vi "Analysis.Selection.Create.vi"(8 "error in (no error)":errorcluster, 9 "Name":string, 10 "Analysis Options":T2, 11 "Item Ref in":T1 format="%.0x") -> (0 "error out":errorcluster)   [LabVIEW 2015, in "Fuel Injection Addon System Explorer.lvlib"]
uses:
  Fuel Injection Addon System Explorer.lvlib
  Shared/Types/Analysis.Channels.Select.ctl
  <vilib>/NI Veristand/Custom Device API/Custom Device Item Ref.ctl
  Shared/Constants.vi
  <vilib>/NI Veristand/Custom Device Tools/Custom Device Utility Library/NI VeriStand - Search for All Items by GUID.vi
  <vilib>/NI VeriStand/Custom Device API/Custom Device API.lvlib
  <vilib>/NI Veristand/Custom Device Tools/Custom Device Utility Library/Custom Device Utility Library.lvlib
  Shared/Fuel Injection Addon Shared.lvlib
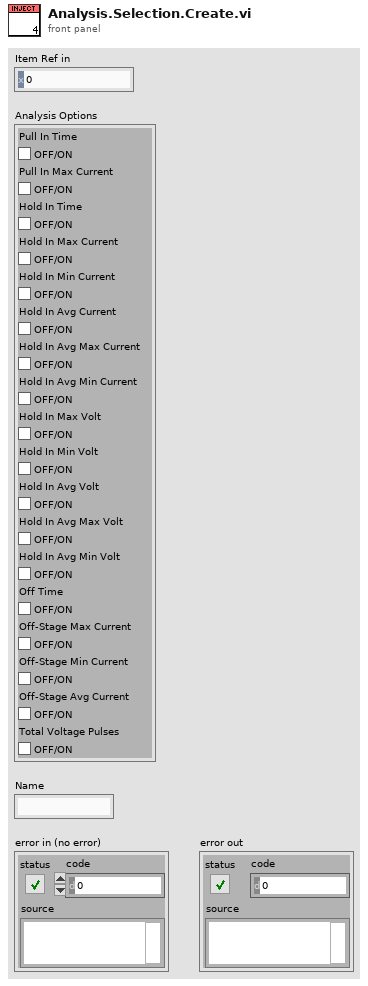
[diagram p1: front panel]
types:
  T1 = typedef "Custom Device API.lvlib/Custom Device Item Ref.ctl" = u64
  T2 = typedef "Fuel Injection Addon Shared.lvlib/Analysis.Channels.Select.ctl" = cluster{"Pull In Time":bool, "Pull In Max Current":bool, "Hold In Time":bool, "Hold In Max Current":bool, "Hold In Min Current":bool, "Hold In Avg Current":bool, "Hold In Avg Max Current":bool, "Hold In Avg Min Current":bool, "Hold In Max Volt":bool, "Hold In Min Volt":bool, "Hold In Avg Volt":bool, "Hold In Avg Max Volt":bool, "Hold In Avg Min Volt":bool, "Off Time":bool, "Off-Stage Max Current":bool, "Off-Stage Min Current":bool, "Off-Stage Avg Current":bool, "Total Voltage Pulses":bool}
  T3 = typedef "Custom Device API.lvlib/Custom Device Item Info.ctl" = cluster{"Name":string, "Is Channel":bool, "GUID":string, "Is Waveform":bool}
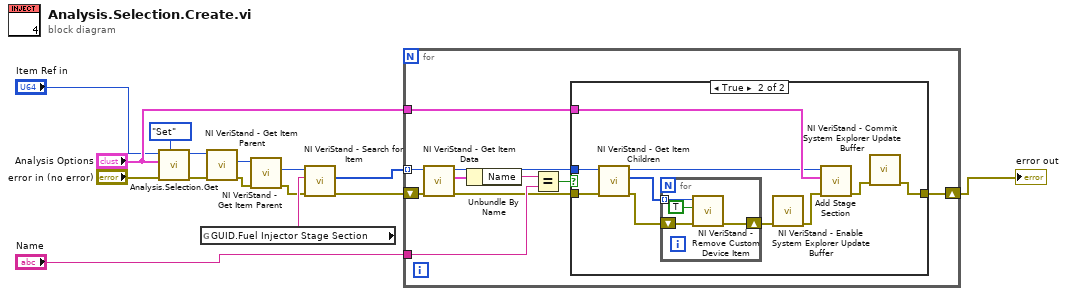
[diagram p0: block diagram]
diagram:
  n1 = call "Analysis.Selection.Get.vi"("Action"=enum8{"Get", "Set"}."Set", "error in (no error)"="error in (no error)", "Selections"="Analysis Options", "Item Ref in"="Item Ref in") -> ("error out"=w12:errorcluster, "Item Ref out"=w11:T1)  [unwired: 5 in, 1 out]
  n2 = global read "Constants.vi" "GUID.Fuel Injector Stage Section"() -> (w5:string)
  n3 = call <vilib>:"NI VeriStand - Get Item Parent.vi"("error in (no error)"=w12, "Item Ref in"=w11) -> ("error out"=w2:errorcluster, "Parent Ref"=w1:T1)  [unwired: 6 in, 2 out]
  n4 = call <vilib>:"NI VeriStand - Get Item Parent.vi"("error in (no error)"=w2, "Item Ref in"=w1) -> ("error out"=w4:errorcluster, "Parent Ref"=w3:T1)  [unwired: 6 in, 2 out]
  n5 = call-poly <vilib>:"NI VeriStand - Search for Item.vi"("error in"=w4, "Item GUID"=w5, "Section Ref in"=w3) -> ("error out"=w8:errorcluster, "Item Refs"=w6:T1[])  [unwired: 5 in, 2 out]
  n6 = for {
    tunnel: w6 -> [w24] mode=indexing
    shift-right: [w16] -> w15
    shift-left: w8 -> [w25]
    tunnel: "Name" -> [w20]
    tunnel: "Analysis Options" -> [w18]
    n7 = call <vilib>:"NI VeriStand - Get Item Data.vi"("error in (no error)"=w25, "Item Ref in"=w24) -> ("error out"=w17:errorcluster, "Item Info"=w22:T3, "Item Ref out"=w23:T1)  [unwired: 6 in, 1 out]
    n8 = Unbundle By Name(w22) -> ("Name"=w21:string)
    n9 = Equal?(x=w21, y=w20) -> (x = y?=w19:bool)
    n10 = case shown="True" w19 {
      tunnel: [w26 w30] -> w16
      tunnel: w23 -> [_ w36]
      tunnel: w18 -> [_ w35]
      tunnel: w17 -> [w26 w27]
      frame False {
      }
      frame True {
        n11 = call <vilib>:"NI VeriStand - Get Item Children.vi"("error in (no error)"=w27, "Item Ref in"=w36) -> ("error out"=w32:errorcluster, "Child Refs"=w33:T1[], "Item Ref out"=w34:T1)  [unwired: 6 in, 1 out]
        n12 = for {
          tunnel: w33 -> [w40] mode=indexing
          shift-right: [w38] -> w29
          shift-left: w32 -> [w39]
          n13 = call <vilib>:"NI VeriStand - Remove Custom Device Item.vi"("error in (no error)"=w39, "Force Delete (F)"=TRUE, "Item Ref in"=w40) -> ("error out"=w38:errorcluster)  [unwired: 7 in, 1 out]
        }
        n14 = call <vilib>:"NI VeriStand - Enable System Explorer Update Buffer.vi"("error in (no error)"=w29) -> ("error out"=w28:errorcluster)  [unwired: 10 in]
        n15 = call "Add Stage Section.vi"("error in (no error)"=w28, "Analysis Options"=w35, "Shot Section reference in"=w34) -> ("error out"=w31:errorcluster)  [unwired: 7 in, 1 out]
        n16 = call <vilib>:"NI VeriStand - Commit System Explorer Update Buffer.vi"("error in (no error)"=w31) -> ("error out"=w30:errorcluster)  [unwired: 10 in]
      }
    }
  }
  "error out" <- w15
